vi "14.-Crear Tablas de Datos.vi"() -> ()   [LabVIEW 2020]
panel:
  out "Table Indicador":string[][](table)
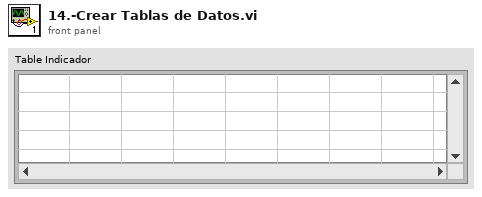
[diagram p1: front panel]
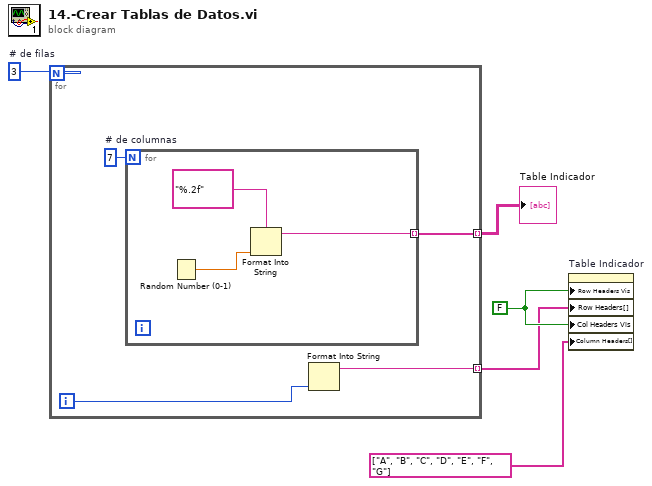
[diagram p0: block diagram]
diagram:
  w3 = FALSE
  w5 = 3  # # de filas
  n1 = for {
    N: w5 -> [_]
    tunnel: [w8] -> w2 mode=indexing
    tunnel: [w6] -> w4 mode=indexing
    i -> [w7]
    w9 = 7  # # de columnas
    n2 = for {
      N: w9 -> [_]
      tunnel: [w10] -> w6 mode=indexing
      n3 = Random Number (0-1)() -> (number: 0 to 1=w12:dbl)
      n4 = Format Into String "Format Into String"(format string="%.2f", w12) -> (resulting string=w10:string)  [unwired: 2 in, 1 out]
    }
    n5 = Format Into String "Format Into String"(w7) -> (resulting string=w8:string)  [unwired: 3 in, 1 out]
  }
  "Table Indicador" <- w4
  n6 = property on="Table Indicador" class="Tbl (strict)"("Row Headers Vis"=w3, "Row Headers[]"=w2, "Col Headers Vis"=w3, "Column Headers[]"=string[] ["A", "B", "C", "D", "E", "F", "G"]) -> ()  [unwired: 2 in, 2 out]
